vi "UpdateDevSP.vi"(7 "LVWSR":refnum<class "Web Request.lvclass">, 10 "sp":dbl, 11 "idx":string) -> ()   [LabVIEW 2017]
uses:
  <vilib>/wsapi/Web Request.lvclass
  Controller/Messages/Update Ctl Device Setpoint MSG/Update Ctl Device Setpoint MSG.lvclass
  C:/Program Files (x86)/National Instruments/LabVIEW 2017/vi.lib/ActorFramework/Message/Message.lvclass
  Controller/Messages/Update Ctl Device Setpoint MSG/Update Ctl Device Setpoint MSG.lvclass/Update Ctl Device Setpoint MSG.ctl
  <vilib>/ActorFramework/Message Enqueuer/Message Enqueuer.lvclass/Message Enqueuer.ctl
  Controller/Messages/Update Ctl Device Setpoint MSG/Write device.vi
  Controller/Messages/Update Ctl Device Setpoint MSG/Write sp.vi
  <vilib>/ActorFramework/Message Priority Queue/Priority Enqueue.vi
  Controller/gController.lvclass
  <vilib>/ActorFramework/Message Enqueuer/Message Enqueuer.lvclass
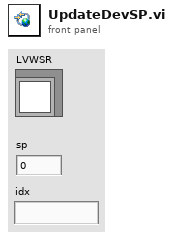
[diagram p1: front panel]
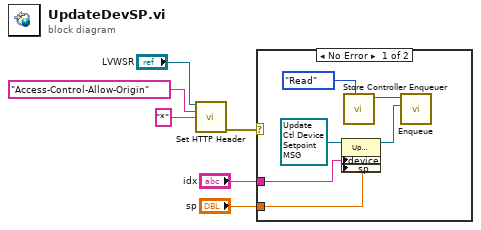
[diagram p0: block diagram]
diagram:
  n1 = call <vilib>:"Set HTTP Header.vi"("LabVIEW Web Service Request"="LVWSR", "header"="Access-Control-Allow-Origin", "header value"="*") -> ("error out"=w3:errorcluster)  [unwired: 11 in, 1 out]
  n2 = case shown="No Error" w3 {
    tunnel: "idx" -> [w10 _]
    tunnel: "sp" -> [w9 _]
    frame No Error {
      n3 = property class="Update Device Setpoint MSG"(reference=refnum<class "Update Ctl Device Setpoint MSG.lvclass"> refnum ("Controller.lvlib:Update Device Setpoint MSG"), "device"=w10, "sp"=w9) -> (reference out=w7:refnum<class "Update Ctl Device Setpoint MSG.lvclass">)  [unwired: 1 in, 1 out]
      n4 = call "Store Controller Enqueuer.vi"("State"=enum16{"Write", "Read"}."Read") -> ("Controller Enqueuer Out"=w8:refnum<class "Message Enqueuer.lvclass">)  [unwired: 10 in]
      n5 = call <vilib>:"Enqueue.vi"("Message"=w7, "Message Enqueuer in"=w8) -> ()  [unwired: 8 in, 2 out]
    }
    frame Error {
    }
  }
